vi "CoboltLaser_DmodEnGet.vi"(8 "ErrorIn":errorcluster, 9 "Mode":T1, 10 "CheckResponse":bool=TRUE, 11 "ComPort":refnum<visa-resource-name>) -> (0 "ErrorOut":errorcluster, 1 "Enabled":bool, 2 "Response":string, 3 "ComPortOut":refnum<visa-resource-name>, 4 "ResponseOK":bool)   [LabVIEW 2019]
doc: "Use this template to build a VI to use as a subVI."
uses:
  Programmes Labview/LabScanV1A/DevicesClass/InstrumentsClass/CoboltMLD/CoboltModes.ctl
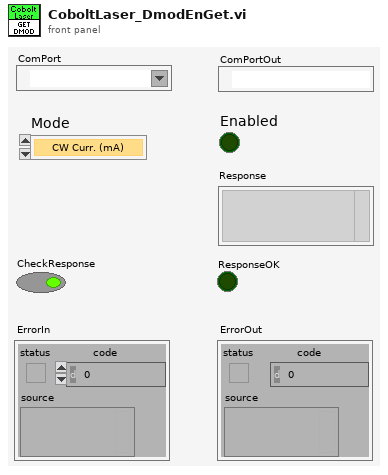
[diagram p1: front panel]
types:
  T1 = typedef "CoboltModes.ctl" = enum16{"CW Curr. (mA)", "CW Pow. (mW)", "Curr. Mod. (mA)", "Pow. Mod. (mW)"}
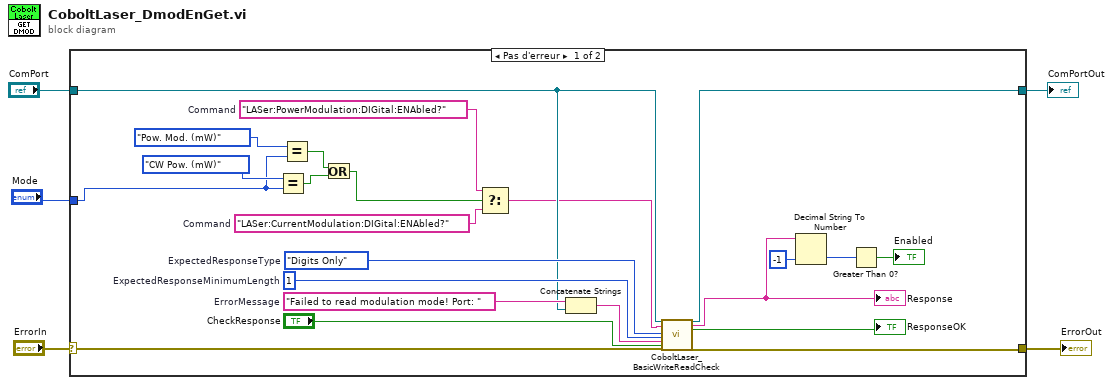
[diagram p0: block diagram]
diagram:
  n1 = case shown="Pas d'erreur" "ErrorIn" {
    selector: "ErrorIn" -> [w28 w30]
    tunnel: [w27 w30] -> w4
    tunnel: "ComPort" -> [w20 w29]
    tunnel: [w19 w29] -> w2
    tunnel: "Mode" -> [w10 _]
    frame No Error {
      w13 = "LASer:CurrentModulation:DIGital:ENAbled?"  # Command
      w14 = "LASer:PowerModulation:DIGital:ENAbled?"  # Command
      w25 = 1  # ExpectedResponseMinimumLength
      w26 = enum16{"Any", "Digits Only", "Non-Digits Only"}."Digits Only"  # ExpectedResponseType
      w22 = "Failed to read modulation mode! Port: "  # ErrorMessage
      n2 = Equal?(x=CoboltModes."CW Pow. (mW)", y=w10) -> (x = y?=w7:bool)
      n3 = Equal?(x=CoboltModes."Pow. Mod. (mW)", y=w10) -> (x = y?=w8:bool)
      n4 = Or(x=w8, y=w7) -> (x .or. y?=w6:bool)
      n5 = Select(t=w14, s=w6, f=w13) -> (s? t:f=w12:string)
      n6 = Concatenate Strings(w22, w20) -> (w21:string)
      n7 = call <userlib>:"CoboltLaser_BasicWriteReadCheck.vi"("ComPort"=w20, "Command"=w12, "ExpectedResponseType"=w26, "ExpectedResponseMinimumLength"=w25, "ErrorMessage"=w21, "GenerateError"="CheckResponse", "error in (no error)"=w28) -> ("ComPortOut"=w19:refnum<visa-resource-name>, "Response"=w18:string, "ResponseOK"=→"ResponseOK":bool, "error out"=w27:errorcluster)  [unwired: 17 in]
      "Response" <- w18
      n8 = Decimal String To Number(string=w18, default (0L)=-1 ("valeur par défaut (0 I32)")) -> (number=w16:i32)  [unwired: 1 in, 1 out]
      n9 = Greater Than 0?(x=w16) -> (x > 0?=→"Enabled":bool)
    }
    frame Error {
    }
  }
  "ErrorOut" <- w4
  "ComPortOut" <- w2
